vi "RestoreFromTaskbar.vi"(8 "error in (no error)":errorcluster, 9 "Show On Taskbar? (T)":bool=TRUE, 10 "VI Refnum":refnum<vi>) -> (0 "error out":errorcluster)   [LabVIEW 2016, in "MGI_TrayIcon.lvclass"]
doc: "Restores a VI what has previously been Minimized to Tray.\n\nIf VI Refnum is unwires, the calling VI will be used.\n\nSet Show on Taskbar? to false to keep the VI from showing in the taskbar.\n\nAuthored by Derek E. Trepanier\nsupport@mooregoodideas.com\nwww.mooregoodideas.com\n\nCopyright (c) 2012, Moore Good Ideas, Inc.\n\nAll rights reserved.\n\nRedistribution and use in source and binary forms, with or without modification, are permitted provided that the following conditions are met:\n\n * Redistributions of source code must retain the above copyright notice, this list of conditions and the following disclaimer.\n * Redistributions in binary form must reproduce the above copyright notice, this list of conditions and the following disclaimer in the documentation and/or other materials provided with the distribution.\n * Neither the name of Moore Good Ideas, Inc. nor the names of its contributors may be used to endorse or promote products derived from this software without specific prior written permission.\n\nTHIS SOFTWARE IS PROVIDED BY THE COPYRIGHT HOLDERS AND CONTRIBUTORS \"AS IS\" AND ANY EXPRESS OR IMPLIED WARRANTIES, INCLUDING, BUT NOT LIMITED TO, THE IMPLIED WARRANTIES OF MERCHANTABILITY AND FITNESS FOR A PARTICULAR PURPOSE ARE DISCLAIMED. IN NO EVENT SHALL THE COPYRIGHT OWNER OR CONTRIBUTORS BE LIABLE FOR ANY DIRECT, INDIRECT, INCIDENTAL, SPECIAL, EXEMPLARY, OR CONSEQUENTIAL DAMAGES (INCLUDING, BUT NOT LIMITED TO, PROCUREMENT OF SUBSTITUTE GOODS OR SERVICES; LOSS OF USE, DATA, OR PROFITS; OR BUSINESS INTERRUPTION) HOWEVER CAUSED AND ON ANY THEORY OF LIABILITY, WHETHER IN CONTRACT, STRICT LIABILITY, OR TORT (INCLUDING NEGLIGENCE OR OTHERWISE) ARISING IN ANY WAY OUT OF THE USE OF THIS SOFTWARE, EVEN IF ADVISED OF THE POSSIBILITY OF SUCH DAMAGE."
uses:
  <userlib>/_MGI/Menu Building/MenuTypes/TrayIcon/MGI_TrayIcon.lvclass
  <userlib>/_MGI/Application Control/MGI VI Reference/MGI Caller's VI Reference.vi
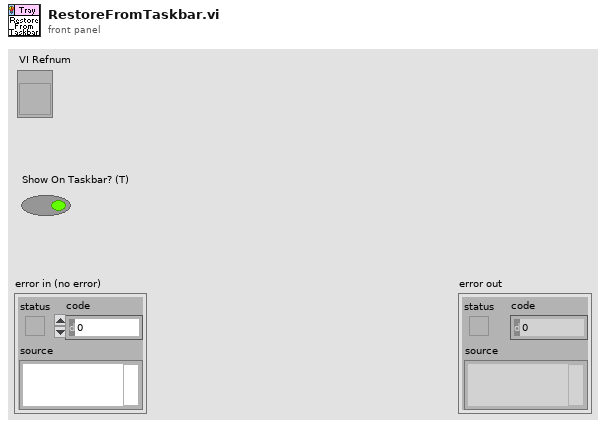
[diagram p1: front panel]
types:
  T1 = enum32{"Invalid", "Standard", "Closed", "Hidden", "Minimized", "Maximized"}
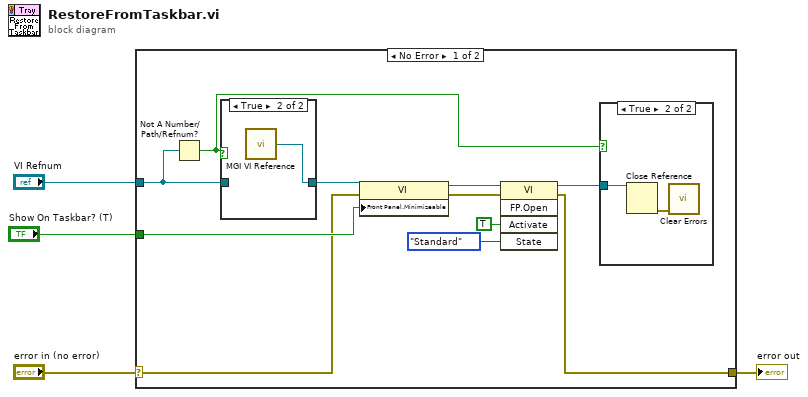
[diagram p0: block diagram]
diagram:
  n1 = case shown="No Error" "error in (no error)" {
    selector: "error in (no error)" -> [w11 w20]
    tunnel: [w9 w20] -> w3
    tunnel: "VI Refnum" -> [w7 _]
    tunnel: "Show On Taskbar? (T)" -> [w12 _]
    frame No Error {
      n2 = Not A Number/Path/Refnum?(number/path/refnum=w7) -> (NaN/Path/Refnum?=w6:bool)
      n3 = case shown="True" w6 {
        tunnel: w7 -> [w18 _]
        tunnel: [w18 w19] -> w8
        frame False {
        }
        frame True {
          n4 = call-poly <userlib>:"MGI VI Reference.vi"() -> ("Caller's VI Reference"=w19:refnum<vi>)  [unwired: 1 in]
        }
      }
      n5 = property class="VI"(reference=w8, error in=w11, "Front Panel.Minimizeable"=w12) -> (reference out=w13:refnum<vi>, error out=w10:errorcluster)
      n6 = invoke class="VI" method="FP.Open"(reference=w13, error in=w10, "Activate"=TRUE ("Activate?"), "State"=T1."Standard") -> (reference out=w5:refnum<vi>, error out=w9:errorcluster)  [unwired: 1 in, 3 out]
      n7 = case shown="True" w6 {
        tunnel: w5 -> [_ w17]
        frame False {
        }
        frame True {
          n8 = Close Reference(reference=w17) -> (error out=w16:errorcluster)  [unwired: 1 in]
          n9 = call <vilib>:"Clear Errors.vi"("error in (no error)"=w16) -> ()  [unwired: 5 in, 2 out]
        }
      }
    }
    frame Error {
    }
  }
  "error out" <- w3
